vi "U6 eAIN Example.vi"() -> (0 "error out":errorcluster)   [LabVIEW 2021]
panel:
  in  "ChannelN":i32=199
  in  "Binary":bool
  in  "AIN Range":u16(ring) items=["LJ_rgBIP10V", "LJ_rgBIP1V", "LJ_rgBIPP1V", "LJ_rgBIPP01V"]
  in  "Resolution":i32
  in  "FirstFound":bool=TRUE
  in  "Address":string="1"
  in  "ChannelP":i32
  out "Error Message":string="No Error"
  out "Value Read":dbl=41420.0 format="%.6f"
  # "Reads 1 analog input using the UD easy function eAIN."
  # "14 = Temp degC\n15 = GND"
  # "15 = Single-Ended\nChannelP+1 = Differential"
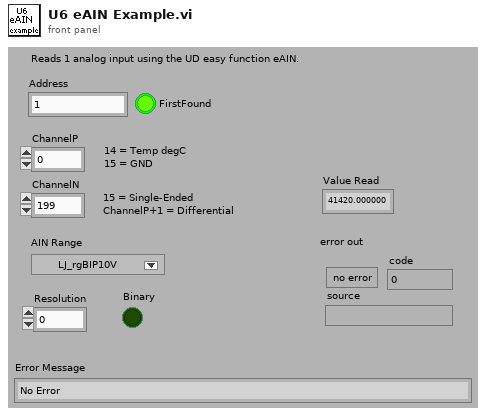
[diagram p1: front panel]
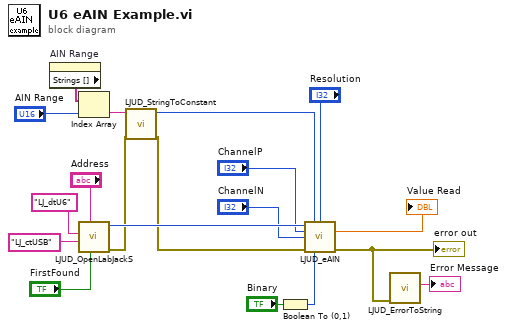
[diagram p0: block diagram]
diagram:
  n1 = property on="AIN Range" class="Ring (strict)"() -> ("Strings []"=w7:string[])  [unwired: 2 in, 2 out]
  n2 = Index Array(array=w7, index="AIN Range") -> (element=w5:string)
  n3 = call "LJUD_OpenLabJackS.vi"("FirstFound"="FirstFound", "Address"="Address", "ConnectionType"="LJ_ctUSB", "DeviceType"="LJ_dtU6") -> ("error out"=w10:errorcluster, "Handle"=w14:i32)  [unwired: 5 in, 1 out]
  n4 = call "LJUD_StringToConstant.vi"("error in"=w10, "String"=w5) -> ("error out"=w9:errorcluster, "Constant Number"=w12:i32)  [unwired: 8 in]
  n5 = Boolean To (0,1)(Boolean="Binary") -> (0, 1=w3:i16)
  n6 = call "LJUD_eAIN.vi"("Handle In"=w14, "Range"=w12, "Resolution"="Resolution", "ChannelP"="ChannelP", "ChannelN"="ChannelN", "error in"=w9, "Binary"=w3) -> ("Voltage"=→"Value Read":dbl, "error out"=w18:errorcluster)  [unwired: 6 in, 1 out]
  "error out" <- w18
  n7 = call "LJUD_ErrorToString.vi"("error in"=w18) -> ("String"=→"Error Message":string)  [unwired: 10 in]
